vi "c ctre phoenixpro Request Control Balance Battery.vi"(7 "cancelOtherRequests":bool, 8 "error in (no error)":errorcluster, 9 "updateTime":dbl, 10 "ecuEncoding":u32, 11 "canbus":string) -> (0 "error out":errorcluster, 3 "function return":i32)   [LabVIEW 2020, in "CTRE_PhoenixTools.lvlib"]
doc: "CTREXPORT int c_ctre_phoenixpro_RequestControlBalanceBattery(const char *canbus, uint32_t ecuEncoding, double updateTime, bool cancelOtherRequests);"
uses:
  CTRE_PhoenixTools.lvlib
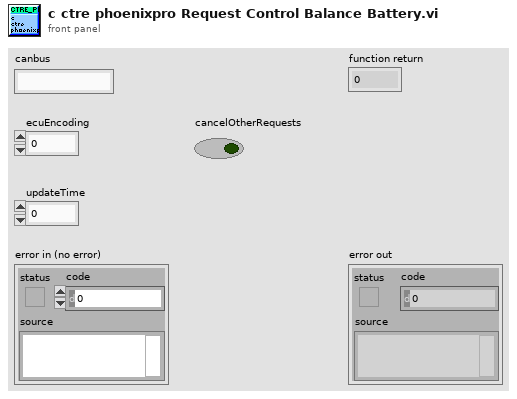
[diagram p1: front panel]
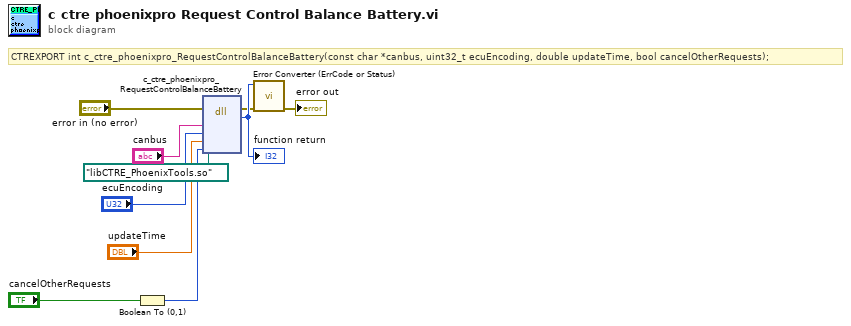
[diagram p0: block diagram]
diagram:
  # "CTREXPORT int c_ctre_phoenixpro_RequestControlBalanceBattery(const char *canbus, uint32_t ecuEncoding, double updateTime, bool cancelOtherRequests);"
  n1 = Boolean To (0,1)(Boolean="cancelOtherRequests") -> (0, 1=w5:i16)
  n2 = dll-call lib="?" fn="c_ctre_phoenixpro_RequestControlBalanceBattery"(path in=path "libCTRE_PhoenixTools.so", error in="error in (no error)", "canbus"="canbus", "ecuEncoding"="ecuEncoding", "updateTime"="updateTime", "cancelOtherRequests"=w5) -> (error out=w3:errorcluster, "return type"=w10:i32)  [unwired: 5 in, 1 out]
  "function return" <- w10
  n3 = call "Error Converter (ErrCode or Status).vi"("error in (no error)"=w3, "error code"=w10) -> ("error out"=→"error out":errorcluster)  [unwired: 9 in]
